vi "tcp_build_packet.vi"(4 "num":u32, 5 "len":u32, 6 "err":u32, 9 "State in":T2, 10 "data":u32[](array[numeric]), 11 "Cmd":T1) -> (3 "tcp_packet":T3)   [LabVIEW 2021]
uses:
  typedefs/tcp_packet.ctl
  typedefs/tcp_cmd.ctl
  typedefs/tcp_states.ctl
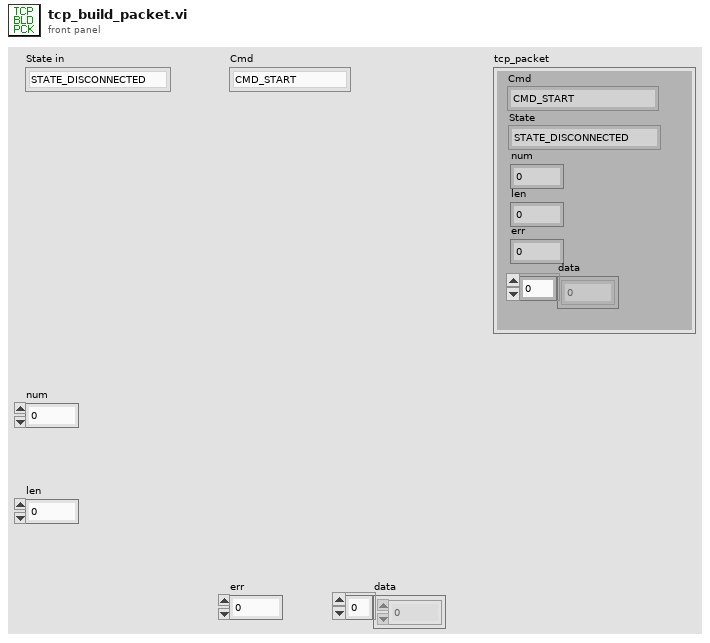
[diagram p1: front panel]
types:
  T1 = typedef "tcp_cmd.ctl" = enum32{"CMD_START", "CMD_SOFTTRIG", "CMD_SETTSET", "CMD_SETTREAD", "CMD_TRANS_START", "CMD_TRANS_LEN", "CMD_TRANS_FINISH"}
  T2 = typedef "tcp_states.ctl" = enum32{"STATE_DISCONNECTED", "STATE_IDLE", "STAIT_WAITINGTRIG", "STATE_ACQUISITION", "STATE_DATARDY", "STATE_DATATRANS", "STATE_ERROR"}
  T3 = typedef "tcp_packet.ctl" = cluster{"Cmd":T1, "State":T2, "num":u32, "len":u32, "err":u32, "data":u32[]}
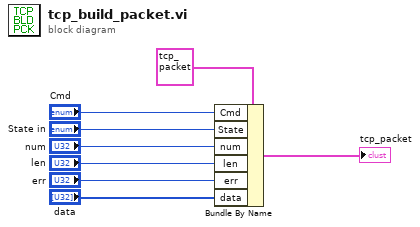
[diagram p0: block diagram]
diagram:
  n1 = Bundle By Name(cluster=T3 {"Cmd"=enum."CMD_START", "State"=enum."STATE_DISCONNECTED", "num"=0, "len"=0, "err"=0, "data"=[]} ("tcp_packet"), "Cmd"="Cmd", "State"="State in", "num"="num", "len"="len", "err"="err", "data"="data") -> (→"tcp_packet":T3)
